vi "Read data.vi"(0 "aNETka config":i32[](array[numeric])=[2, 5, 1], 4 "Data file path":path) -> (7 "Up Targets":sgl[](array[numeric])=[13.735858] format="%.2f", 8 "Inputs":string[](array[string])=["Input 1", "Input 2"], 9 "Down Targets":sgl[](array[numeric])=[-8.885134] format="%.2f", 10 "Targets":string[](array[string])=["Output 1"], 11 "Up Inputs":sgl[](array[numeric])=[511.0, 11.026564] format="%.2f", 12 "Continue? (T=yes)":bool=TRUE, 13 "Down Inputs":sgl[](array[numeric])=[1.0, 20.0] format="%.2f", 14 "Scaled inputs":sgl[][](array[numeric])=[[0.05, 0.05], [0.051761255, 0.13162108], [0.05528376, 0.21732314], [0.062328767, 0.30731046], [0.07641879, 0.4017971], [0.10459883, 0.5010079], [0.1609589, 0.60517937], [0.27367905, 0.71455944], [0.49911937, 0.8294085], [0.95, 0.95]] format="%.2f", 15 "Scaled targets":sgl[][](array[numeric])=[[0.70459014], [0.7114872], [0.72673327], [0.76687974], [0.95000005], [0.05], [0.4722297], [0.5297184], [0.5495496], [0.5581958]] format="%.2f", 18 "Inputs":sgl[][](array[numeric])=[[1.0, 20.0], [2.0, 21.0], [4.0, 22.05], [8.0, 23.1525], [16.0, 24.310125], [32.0, 25.52563], [64.0, 26.801912], [128.0, 28.142008], [256.0, 29.549109], [512.0, 31.026564]] format="%.2f", 19 "Targets":sgl[][](array[numeric])=[[1.1052631], [1.2105263], [1.4432133], [2.0559313], [4.850724], [-8.885134], [-2.4410372], [-1.5636406], [-1.2609758], [-1.1290157]] format="%.2f")   [LabVIEW 2010]
uses:
  <vilib>/Utility/file.llb/Read From Spreadsheet File (DBL).vi
panel:
  in  "OK":bool
  in  "Exit":bool
  in  "Targets start at column\n(type number from first row below)":i32=2 min=0 max=1000
  in  "Inputs start at column \n(type number from first row below)":i32 min=0 max=1000 step=1
  out "Column nr":i32[](array[numeric])=[0, 1, 2]
  out "Column\ncaptions":string[](array[string])=["Input 1", "Input 2", "Output 1"]
  out "Data":sgl[][](array[numeric])=[[1.0, 20.0, 1.1052631], [2.0, 21.0, 1.2105263], [4.0, 22.05, 1.4432133], [8.0, 23.1525, 2.0559313], [16.0, 24.310125, 4.850724], [32.0, 25.52563, -8.885134], [64.0, 26.801912, -2.4410372], [128.0, 28.142008, -1.5636406], [256.0, 29.549109, -1.2609758], [512.0, 31.026564, -1.1290157]] step=0.05 format="%.2f"
  # "Rows\nColumns"
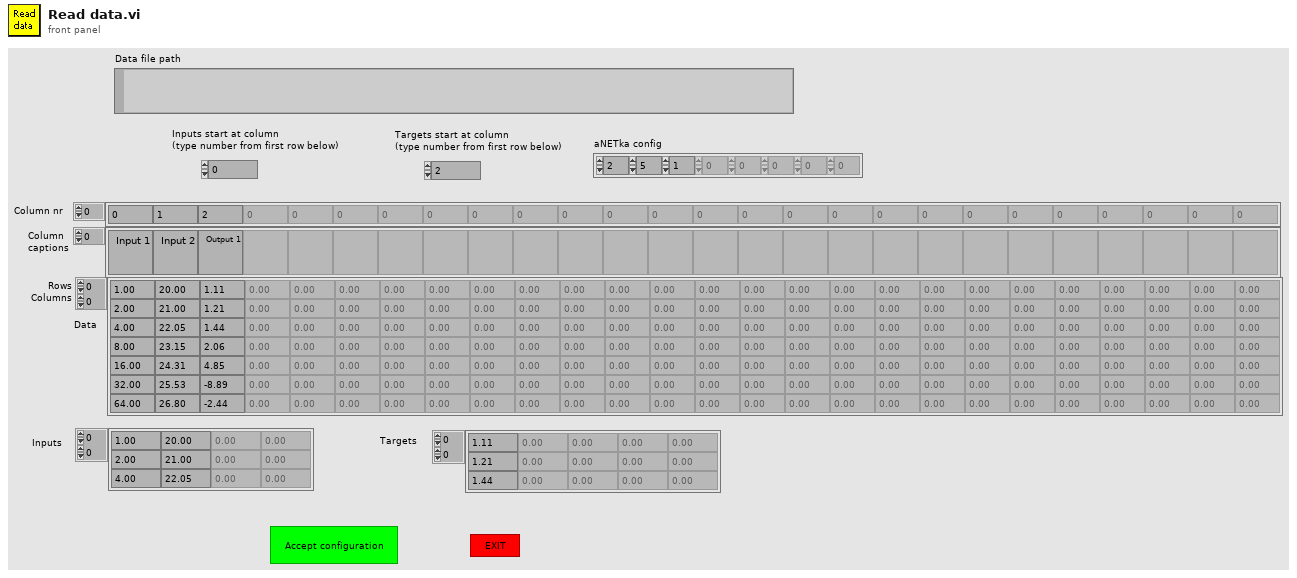
[diagram p1: front panel]
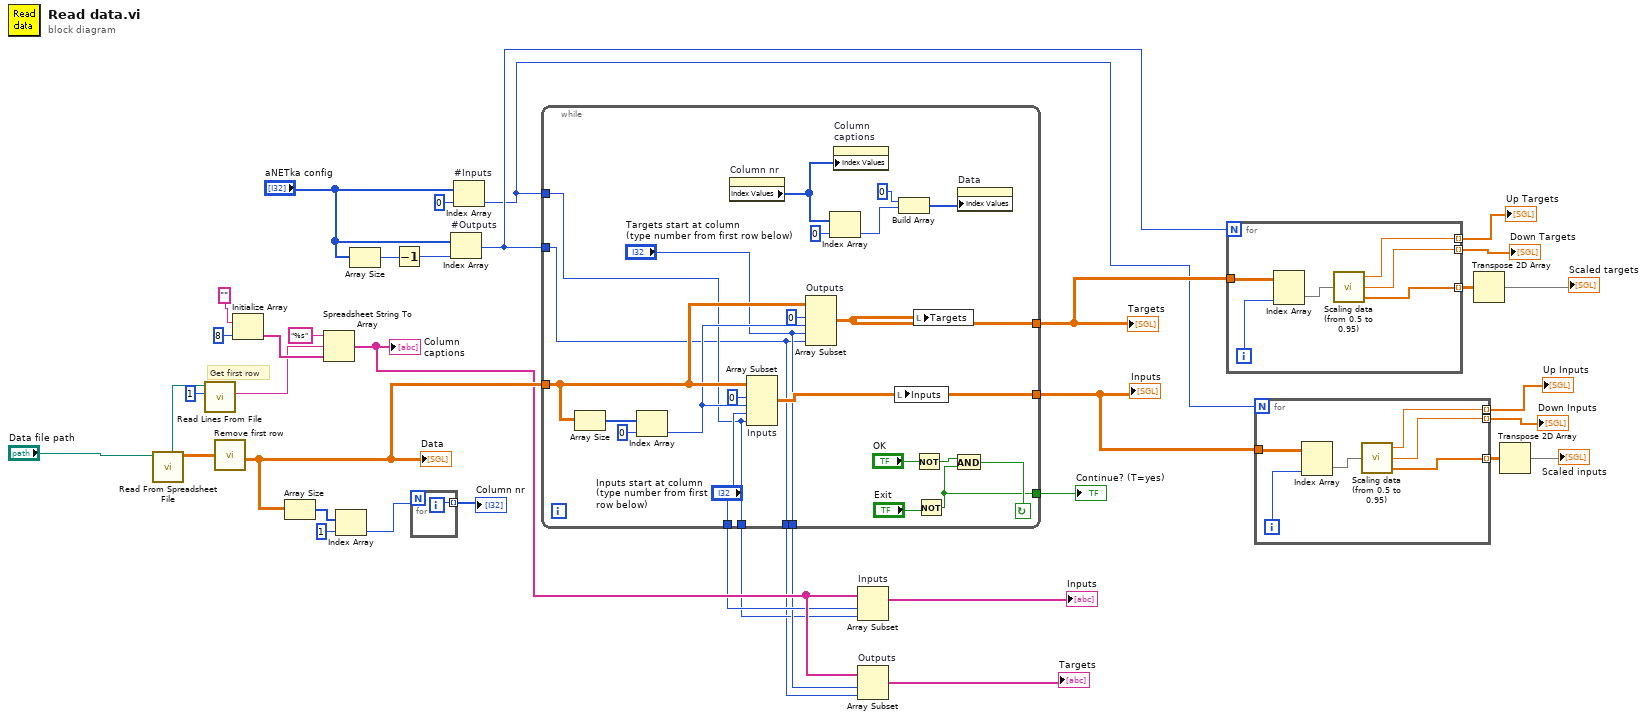
[diagram p0: block diagram]
diagram:
  # "Get first row"
  n1 = call-poly <vilib>:"Read From Spreadsheet File.vi"("file path (dialog if empty)"="Data file path") -> ("all rows"=w32:dbl[][], "new file path (Not A Path if cancelled)"=w31:path)  [unwired: 6 in, 3 out]
  n2 = call <vilib>:"Read Lines From File.vi"("file path (dialog if empty)"=w31, "number of lines (all:-1)"=1) -> ("line string"=w33:string)  [unwired: 4 in, 3 out]
  n3 = call "Remove first row.vi"("Data with comments\nin first row"=w32) -> ("The same data\nwithout first raw"=w24:sgl[][])
  "Data" <- w24
  n4 = Initialize Array("", 8 ("Dimension Size")) -> (w36:string[])
  n5 = Array Size(array=w24) -> (size(s)=w30:i32[])
  n6 = Spreadsheet String To Array(format string="%s", spreadsheet string=w33, array type (2D Dbl)=w36) -> (array=w7:string[])  [unwired: 1 in]
  "Column\ncaptions" <- w7
  n7 = Index Array(array=w30, index=1 ("Index")) -> (element=w28:i32)
  n8 = Array Size(array="aNETka config") -> (size(s)=w21:i32)
  n9 = Decrement(x=w21) -> (x-1=w20:i32)
  n10 = for {
    N: w28 -> [_]
    tunnel: [w39] -> w27 mode=indexing
    i -> [w39]
  }
  "Column nr" <- w27
  n11 = Index Array "#Outputs"(array="aNETka config", index=w20) -> (element=w13:i32)
  n12 = Index Array "#Inputs"(array="aNETka config", index=0 ("Index")) -> (element=w12:i32)
  n13 = while {
    tunnel: [w40] -> w3
    tunnel: [w41] -> w4
    tunnel: ["Targets start at column\n(type number from first row below)"] -> w5
    tunnel: ["Inputs start at column \n(type number from first row below)"] -> w6
    tunnel: [w44] -> w16
    tunnel: [w45] -> w19
    tunnel: w13 -> [w40]
    tunnel: w12 -> [w41]
    tunnel: w24 -> [w48]
    tunnel: [w57] -> w25
    stop <- w58 continue-if-true
    n14 = Array Size(array=w48) -> (size(s)=w42:i32[])
    n15 = Index Array(array=w42, index=0 ("Index")) -> (element=w46:i32)
    n16 = property on="Column nr" class="Arr (strict)"() -> ("Index Values"=w55:u32[])  [unwired: 2 in, 2 out]
    n17 = Array Subset "Inputs"(array=w48, index (row)=0 ("Array Index"), length (row)=w46, index (col)="Inputs start at column \n(type number from first row below)", length (col)=w41) -> (w44:sgl[][])
    n18 = Array Subset "Outputs"(array=w48, index (row)=0 ("Array Index"), length (row)=w46, index (col)="Targets start at column\n(type number from first row below)", length (col)=w40) -> (w45:sgl[][])
    n19 = Index Array(array=w55, index=0 ("Index")) -> (element=w54:u32)
    n20 = property on="Column\ncaptions" class="Arr (strict)"("Index Values"=w55) -> ()  [unwired: 2 in, 2 out]
    n21 = local write "Inputs"(w44) -> ()
    n22 = Build Array(0, w54) -> (w56:u32[])
    n23 = local write "Targets"(w45) -> ()
    n24 = Not(x="OK") -> (.not. x?=w60:bool)
    n25 = Not(x="Exit") -> (.not. x?=w57:bool)
    n26 = And(x=w60, y=w57) -> (x .and. y?=w58:bool)
    n27 = property on="Data" class="Arr (strict)"("Index Values"=w56) -> ()  [unwired: 2 in, 2 out]
  }
  "Continue? (T=yes)" <- w25
  "Targets" <- w19
  "Inputs" <- w16
  n28 = Array Subset "Inputs"(array=w7, index=w6, length=w4) -> (→"Inputs":string[])
  n29 = Array Subset "Outputs"(array=w7, index=w5, length=w3) -> (→"Targets":string[])
  n30 = for {
    N: w13 -> [_]
    tunnel: w19 -> [w66]
    tunnel: [w64] -> w18 mode=indexing
    tunnel: [w63] -> w11 mode=indexing
    tunnel: [w62] -> w10 mode=indexing
    i -> [w67]
    n31 = Index Array(array=w66, index (col)=w67) -> (element=w65:sgl[])  [unwired: 1 in]
    n32 = call "Scaling data (from 0.5 to 0.95).vi"("Input data"=w65) -> ("Offset up"=w63:sgl, "Offset down"=w62:sgl, "Scaled data"=w64:sgl[])
  }
  "Up Targets" <- w11
  "Down Targets" <- w10
  n33 = for {
    N: w12 -> [_]
    tunnel: w16 -> [w72]
    tunnel: [w70] -> w17 mode=indexing
    tunnel: [w69] -> w9 mode=indexing
    tunnel: [w68] -> w8 mode=indexing
    i -> [w73]
    n34 = Index Array(array=w72, index (col)=w73) -> (element=w71:sgl[])  [unwired: 1 in]
    n35 = call "Scaling data (from 0.5 to 0.95).vi"("Input data"=w71) -> ("Offset up"=w69:sgl, "Offset down"=w68:sgl, "Scaled data"=w70:sgl[])
  }
  "Up Inputs" <- w9
  "Down Inputs" <- w8
  n36 = Transpose 2D Array(2D array=w18) -> (transposed array=→"Scaled targets":sgl[][])
  n37 = Transpose 2D Array(2D array=w17) -> (transposed array=→"Scaled inputs":sgl[][])
